vi "ics-http.vi"() -> ()   [LabVIEW 2014]
uses:
  <vilib>/LVH/i3 JSON/JSON Parsing/Get Object Parameter Files/Get Object Parameter - String.vi
  <vilib>/addons/_JKI.lib/REST Client/classes/REST Client/REST Client.lvclass
  <vilib>/LVH/i3 JSON/i3-json.lvlib
panel:
  out "Response body 2":string
  out "Status String":string
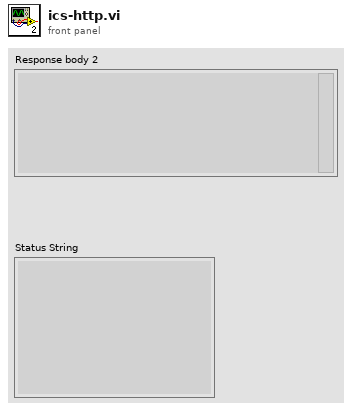
[diagram p1: front panel]
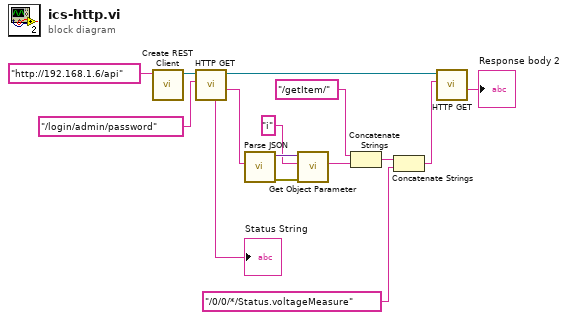
[diagram p0: block diagram]
diagram:
  n1 = call <vilib>:"Create REST Client.vi"("Base URL"="http://192.168.1.6/api") -> ("REST Client out"=w14:refnum<class "REST Client.lvclass">)  [unwired: 9 in, 1 out]
  n2 = call-dynamic "HTTP GET.vi"("Path"="/login/admin/password", "REST Client in"=w14) -> ("Response body"=w11:string, "REST Client out"=w1:refnum<class "REST Client.lvclass">, "Status String"=→"Status String":string)  [unwired: 4 in, 3 out]
  n3 = call <vilib>:"Parse JSON.vi"("JSON String"=w11) -> ("error out"=w10:errorcluster, "JSON Tree"=w9:variant)  [unwired: 7 in, 2 out]
  n4 = call-poly <vilib>:"Get Object Parameter.vi"("error in (no error)"=w10, "Parameter Name"="i", "JSON Tree In (JSON Object)"=w9) -> ("String Value"=w6:string)  [unwired: 5 in, 3 out]
  n5 = Concatenate Strings("/getItem/" ("Path"), w6) -> (w4:string)
  n6 = Concatenate Strings(w4, "/0/0/*/Status.voltageMeasure" ("string")) -> (w3:string)
  n7 = call-dynamic "HTTP GET.vi"("Path"=w3, "REST Client in"=w1) -> ("Response body"=→"Response body 2":string)  [unwired: 4 in, 5 out]
